vi "Логи_ШИМ.vi"() -> ()   [LabVIEW 2013]
panel:
  in  "Tab Control":enum32{"Выходы на моторы", "Частота ШИМ"}(tab)
  out "XY Graph":cluster{dbl[], u16[]}[](graph)
  out "HZ":cluster{dbl[], dbl[]}[](graph)
  out "ID параметров":u8[](array[numeric])
  out "Длина заголовка":i32
  out "Заголовок":string
  out "Количество параметров":u8
  out "size (in bytes)":i64
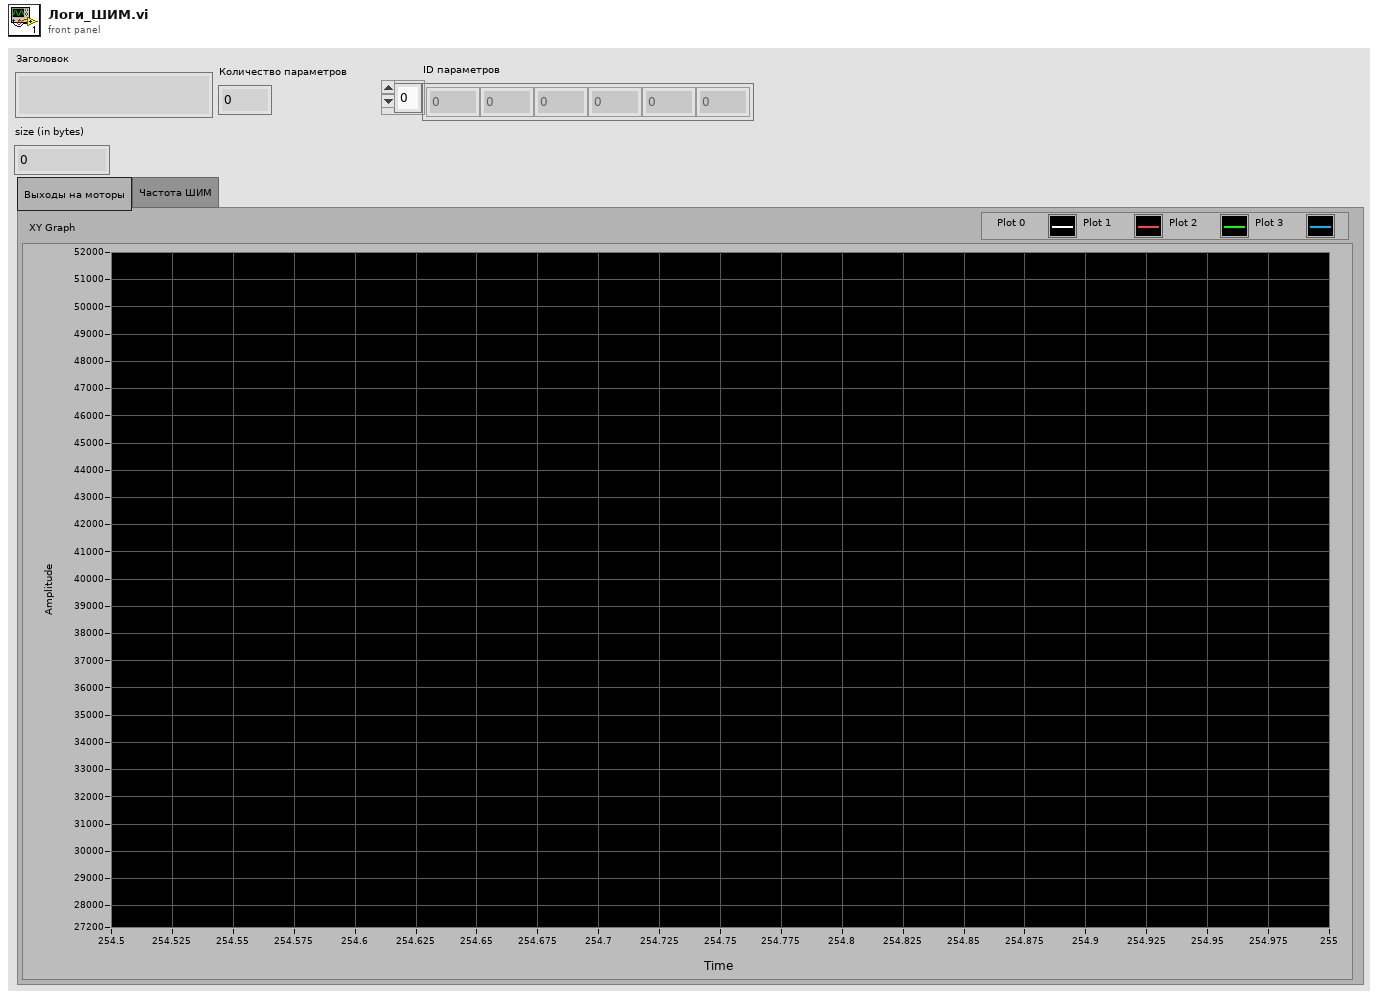
[diagram p1: front panel]
types:
  T1 = enum16{"open", "replace", "create", "open or create", "replace or create", "replace or create with confirmation"}
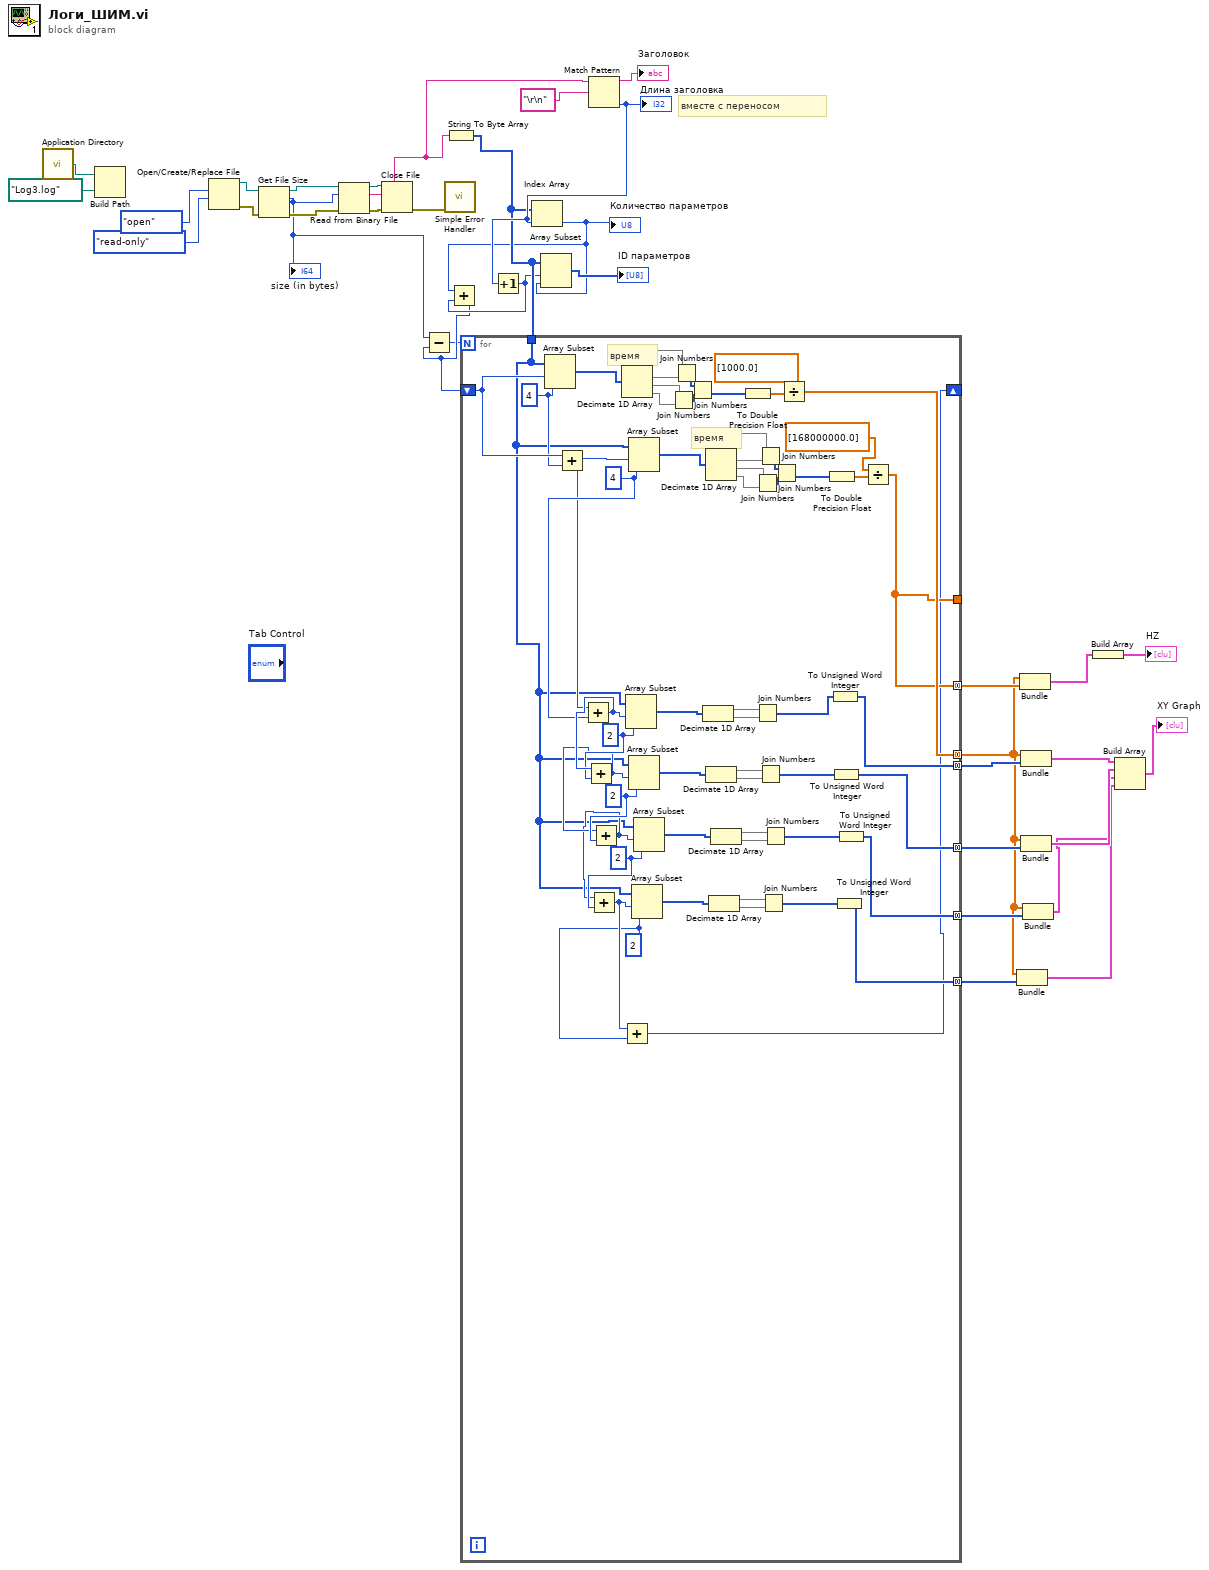
[diagram p0: block diagram]
diagram:
  # "вместе с переносом"
  n1 = call <vilib>:"Application Directory.vi"() -> ("Application Directory"=w32:path)
  n2 = Build Path(base path=w32, name or relative path=path "Log3.log" ("default name")) -> ()  [unwired: 1 out]
  n3 = Open/Create/Replace File(operation (0:open)=T1."open", access (0:read/write)=enum16{"read/write", "read-only", "write-only"}."read-only") -> (refnum out=w29:refnum<file>, error out=w27:errorcluster)  [unwired: 4 in, 1 out]
  n4 = Get File Size(file=w29, error in=w27) -> (refnum out=w28:refnum<file>, size (in bytes)=w19:i64, 0:w26:errorcluster)
  "size (in bytes)" <- w19
  n5 = Read from Binary File(8:w26, 10:w19, 11:w28) -> (0:w30:errorcluster, 2:w25:string, 3:w31:refnum<file>)  [unwired: 3 in, 1 out]
  n6 = Close File(refnum=w31, error in=w30) -> (error out=w35:errorcluster)  [unwired: 1 out]
  n7 = call <vilib>:"Simple Error Handler.vi"("error in (no error)"=w35) -> ()  [unwired: 4 in, 5 out]
  n8 = String To Byte Array(string=w25) -> (unsigned byte array=w20:u8[])
  n9 = Match Pattern(string=w25, regular expression="\r\n" ("format string")) -> (before substring=→"Заголовок":string, offset past match=w22:i32)  [unwired: 1 in, 2 out]
  "Длина заголовка" <- w22
  n10 = Increment(x=w22) -> (x+1=w17:i32)
  n11 = Index Array(array=w20, index=w22) -> (element=w18:u8)
  "Количество параметров" <- w18
  n12 = Add(x=w18, y=w17) -> (x+y=w16:i32)
  n13 = Subtract(x=w19, y=w16) -> (x-y=w15:i64)
  n14 = for {
    N: w15 -> [_]
    tunnel: w20 -> [w39]
    shift-right: [w38] -> _
    shift-left: w16 -> [w46]
    tunnel: [w59] -> w3 mode=concatenating
    tunnel: [w58] -> w9 mode=concatenating
    tunnel: [w57] -> w8 mode=concatenating
    tunnel: [w56] -> w7 mode=concatenating
    tunnel: [w55] -> w6 mode=concatenating
    tunnel: [w40] -> w4 mode=concatenating
    tunnel: [w40] -> _
    w44 = 4 ("length")
    w36 = 2 ("length")
    w70 = 2 ("length")
    w71 = 2 ("length")
    w78 = 2 ("length")
    w45 = 4 ("length")
    # "время"
    # "время"
    n15 = Array Subset(array=w39, index=w46, length=w45) -> (w85:u8[])
    n16 = Add(x=w46, y=w45) -> (x+y=w43:i32)
    n17 = Add(x=w43, y=w44) -> (x+y=w79:i32)
    n18 = Add(x=w79, y=w78) -> (x+y=w69:i32)
    n19 = Add(x=w69, y=w71) -> (x+y=w68:i32)
    n20 = Add(x=w68, y=w70) -> (x+y=w37:i32)
    n21 = Decimate 1D Array(w85) -> (w87:u8[], w88:u8[], w89:u8[], w90:u8[])
    n22 = Add(x=w37, y=w36) -> (x+y=w38:i32)
    n23 = Array Subset(array=w39, index=w79, length=w78) -> (w81:u8[])
    n24 = Array Subset(array=w39, index=w43, length=w44) -> (w48:u8[])
    n25 = Array Subset(array=w39, index=w69, length=w71) -> (w80:u8[])
    n26 = Array Subset(array=w39, index=w37, length=w36) -> (w73:u8[])
    n27 = Array Subset(array=w39, index=w68, length=w70) -> (w75:u8[])
    n28 = Join Numbers(hi=w89, lo=w90) -> ((hi.lo)=w86:u16[])
    n29 = Join Numbers(hi=w87, lo=w88) -> ((hi.lo)=w91:u16[])
    n30 = Join Numbers(hi=w91, lo=w86) -> ((hi.lo)=w82:u32[])
    n31 = Decimate 1D Array(w81) -> (w67:u8[], w66:u8[])
    n32 = Decimate 1D Array(w48) -> (w50:u8[], w51:u8[], w52:u8[], w53:u8[])
    n33 = Decimate 1D Array(w80) -> (w65:u8[], w64:u8[])
    n34 = Decimate 1D Array(w73) -> (w61:u8[], w60:u8[])
    n35 = Decimate 1D Array(w75) -> (w62:u8[], w63:u8[])
    n36 = To Double Precision Float(number=w82) -> (double precision float=w84:dbl[])
    n37 = Join Numbers(hi=w52, lo=w53) -> ((hi.lo)=w49:u16[])
    n38 = Join Numbers(hi=w67, lo=w66) -> ((hi.lo)=w76:u16[])
    n39 = Join Numbers(hi=w50, lo=w51) -> ((hi.lo)=w54:u16[])
    n40 = Join Numbers(hi=w65, lo=w64) -> ((hi.lo)=w77:u16[])
    n41 = Join Numbers(hi=w61, lo=w60) -> ((hi.lo)=w72:u16[])
    n42 = Join Numbers(hi=w62, lo=w63) -> ((hi.lo)=w74:u16[])
    n43 = Join Numbers(hi=w54, lo=w49) -> ((hi.lo)=w47:u32[])
    n44 = Divide(x=w84, y=dbl[] [1000.0]) -> (x/y=w59:dbl[])
    n45 = To Double Precision Float(number=w47) -> (double precision float=w42:dbl[])
    n46 = To Unsigned Word Integer(number=w76) -> (unsigned 16bit integer=w58:u16[])
    n47 = To Unsigned Word Integer(number=w77) -> (unsigned 16bit integer=w57:u16[])
    n48 = To Unsigned Word Integer(number=w72) -> (unsigned 16bit integer=w55:u16[])
    n49 = To Unsigned Word Integer(number=w74) -> (unsigned 16bit integer=w56:u16[])
    n50 = Divide(x=dbl[] [168000000.0] ("y"), y=w42) -> (x/y=w40:dbl[])
  }
  n51 = Array Subset(array=w20, index=w17, length=w18) -> (→"ID параметров":u8[])
  n52 = Bundle(w3, w6) -> (w11:cluster{dbl[], u16[]})  [unwired: 1 in]
  n53 = Bundle(w3, w4) -> (w2:cluster{dbl[], dbl[]})  [unwired: 1 in]
  n54 = Bundle(w3, w9) -> (w14:cluster{dbl[], u16[]})  [unwired: 1 in]
  n55 = Bundle(w3, w8) -> (w13:cluster{dbl[], u16[]})  [unwired: 1 in]
  n56 = Bundle(w3, w7) -> (w12:cluster{dbl[], u16[]})  [unwired: 1 in]
  n57 = Build Array(w2) -> (→"HZ":cluster{dbl[], dbl[]}[])
  n58 = Build Array(w14, w13, w12, w11) -> (→"XY Graph":cluster{dbl[], u16[]}[])
